vi "Level 3 Climb.vi"() -> ()   [LabVIEW 2018]
uses:
  <vilib>/Rock Robotics/WPI/ThirdParty/Phoenix-LabVIEW/Motor Controller/Controls/CTRE_Phoenix_MotorControl_ControlMode.ctl
  <vilib>/Rock Robotics/WPI/ThirdParty/Phoenix-LabVIEW/Motor Controller/Get/CTRE_Phoenix_MotorController_GetSelectedSensorData.vi
panel:
  in  "Boolean":bool
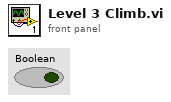
[diagram p1: front panel]
types:
  T1 = typedef "CTRE_Phoenix_MotorControl_ControlMode.ctl" = u16
  T2 = typedef "WPI_MotorControlDeviceRef.ctl" = cluster{"DeviceStatus":errorcluster, "Type":T3, "PWM":cluster{"PWM Channel":T4, "DeadBand":T5}, "CAN":cluster{"Device Number":u8, "SetOutput VI Ref":variant, "GetOutput VI Ref":variant, "Enable VI Ref":variant, "Disable VI Ref":variant, "Data":variant}, "Invert":bool, "DIO PWM":cluster{"PWM \"Enable\" Channel":T4, "DIOChannel":T6, "PWM Rate":dbl}}
  T3 = typedef "WPI_MotorControlType.ctl" = enum16{"PWM", "CAN", "DIO PWM"}
  T4 = typedef "FPGA_DIOPWMChannel.ctl" = enum8{"PWM 0", "PWM 1", "PWM 2", "PWM 3", "PWM 4", "PWM 5", "PWM 6", "PWM 7", "PWM 8", "PWM 9", "PWM MXP 0", "PWM MXP 1", "PWM MXP 2", "PWM MXP 3", "PWM MXP 4", "PWM MXP 5", "PWM MXP 6", "PWM MXP 7", "PWM MXP 8", "PWM MXP 9", "Invalid"}
  T5 = typedef "WPI_PWMDeadband.ctl" = cluster{"Name":string, "maxPositivePwm":i32, "minPositivePwm":i32, "centerPwm":i32, "maxNegativePwm":i32, "minNegativePwm":i32, "angularRange":u16}
  T6 = typedef "FPGA_DIOChannel.ctl" = enum8{"DIO 0", "DIO 1", "DIO 2", "DIO 3", "DIO 4", "DIO 5", "DIO 6", "DIO 7", "DIO 8", "DIO 9", "DIO MXP 0", "DIO MXP 1", "DIO MXP 2", "DIO MXP 3", "DIO MXP 4", "DIO MXP 5", "DIO MXP 6", "DIO MXP 7", "DIO MXP 8", "DIO MXP 9", "DIO MXP 10", "DIO MXP 11", "DIO MXP 12", "DIO MXP 13", "DIO MXP 14", "DIO MXP 15", "SPI Port CS1", "SPI Port CS2", "SPI Port CS3", "SPI Port MISO", "SPI Port MOSI", "Invalid"}
  T7 = typedef "WPI_SwitchDevRef.ctl" = cluster{"DevStatus":errorcluster, "DIO Channel":T6, "CntIndex":T8, "Normally Closed":bool}
  T8 = typedef "FPGA_CounterCtrSystemIndex.ctl" = enum8{"Ctr 0", "Ctr 1", "Ctr 2", "Ctr 3", "Ctr 4", "Ctr 5", "Ctr 6", "Ctr 7", "Invalid"}
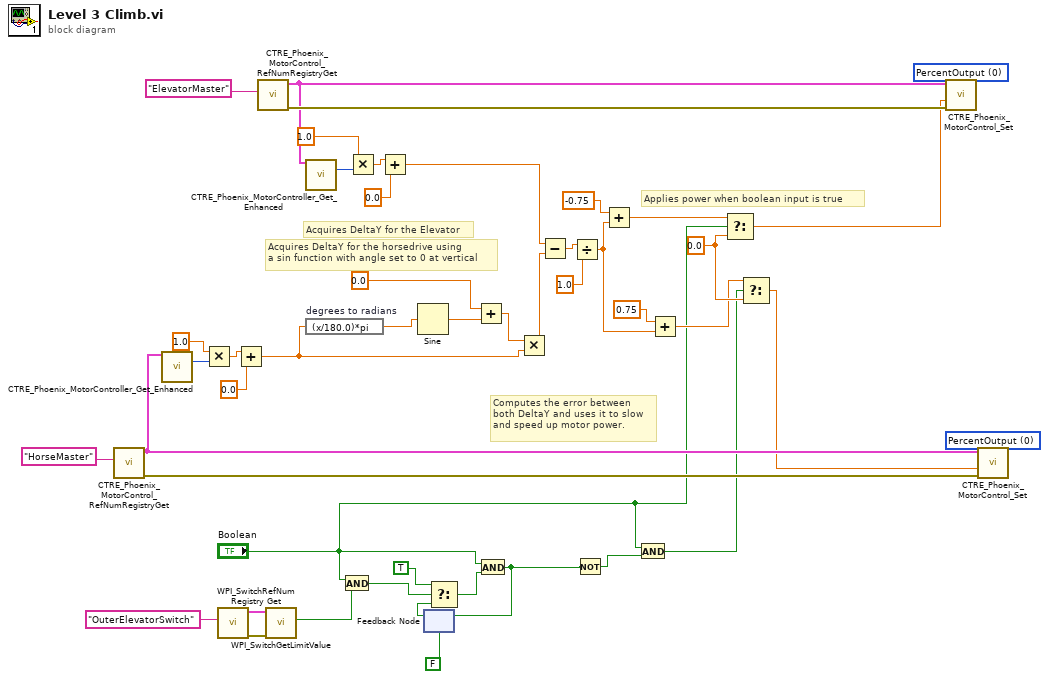
[diagram p0: block diagram]
diagram:
  w42 = T1 0 items=["PercentOutput"=0, "Position"=1, "Velocity"=2, "Current"=3, "Follower"=5, "MotionProfile"=6, "MotionMagic"=7, "MotionProfileArc"=10, "Disabled"=15] ("Control Mode")
  w38 = 0.0 ("f")
  w45 = T1 0 items=["PercentOutput"=0, "Position"=1, "Velocity"=2, "Current"=3, "Follower"=5, "MotionProfile"=6, "MotionMagic"=7, "MotionProfileArc"=10, "Disabled"=15] ("Control Mode")
  # "Applies power when boolean input is true"
  # "Computes the error between\nboth DeltaY and uses it to slow\nand speed up motor power."
  # "Acquires DeltaY for the horsedrive using\na sin function with angle set to 0 at vertical"
  # "Acquires DeltaY for the Elevator"
  n1 = call <vilib>:"CTRE_Phoenix_MotorControl_RefNumRegistryGet.vi"("refnum name"="HorseMaster") -> ("error out"=w41:errorcluster, "PhoenixMotorControlDevRef"=w40:T2)  [unwired: 9 in]
  n2 = call-poly <vilib>:"CTRE_Phoenix_MotorController_Get_Enhanced.vi"("PhoenixMotorControlDevRef"=w40) -> ("Position (Raw Sensor Units)"=w25:i32)  [unwired: 11 in, 3 out]
  n3 = Multiply(x=1.0, y=w25) -> (x*y=w39:dbl)
  n4 = call <vilib>:"WPI_SwitchRefNum Registry Get.vi"("refnum name"="OuterElevatorSwitch") -> ("error out"=w12:errorcluster, "SwitchDevRef"=w11:T7)  [unwired: 9 in]
  n5 = Add(x=w39, y=0.0) -> (x+y=w19:dbl)
  n6 = call <vilib>:"CTRE_Phoenix_MotorControl_RefNumRegistryGet.vi"("refnum name"="ElevatorMaster") -> ("error out"=w46:errorcluster, "PhoenixMotorControlDevRef"=w35:T2)  [unwired: 9 in]
  n7 = call <vilib>:"WPI_SwitchGetLimitValue.vi"("error in (no error)"=w12, "SwitchDevRef"=w11) -> ("Switch Pressed"=w10:bool)  [unwired: 7 in, 2 out]
  n8 = call-poly <vilib>:"CTRE_Phoenix_MotorController_Get_Enhanced.vi"("PhoenixMotorControlDevRef"=w35) -> ("Position (Raw Sensor Units)"=w36:i32)  [unwired: 11 in, 3 out]
  n9 = expression code="(x/180.0)*pi" "degrees to radians"(w19) -> (w21:dbl)
  n10 = And(x="Boolean", y=w10) -> (x .and. y?=w9:bool)
  n11 = Multiply(x=1.0, y=w36) -> (x*y=w37:dbl)
  n12 = Add(x=w37, y=0.0) -> (x+y=w34:dbl)
  n13 = Sine(x=w21) -> (sin(x)=w23:dbl)
  n14 = feedback #1(FALSE) -> (w7:bool)
  n15 = Select(t=TRUE, s=w9, f=w7) -> (s? t:f=w5:bool)
  n16 = Add(x=0.0, y=w23) -> (x+y=w20:dbl)
  n17 = And(x="Boolean", y=w5) -> (x .and. y?=w3:bool)
  n18 = feedback-in #1(w3) -> ()
  n19 = Multiply(x=w20, y=w19) -> (x*y=w24:dbl)
  n20 = Subtract(x=w34, y=w24) -> (x-y=w33:dbl)
  n21 = Divide(x=w33, y=1.0) -> (x/y=w29:dbl)
  n22 = Not(x=w3) -> (.not. x?=w2:bool)
  n23 = Add(x=-0.75, y=w29) -> (x+y=w31:dbl)
  n24 = And(x="Boolean", y=w2) -> (x .and. y?=w1:bool)
  n25 = Add(x=0.75, y=w29) -> (x+y=w28:dbl)
  n26 = Select(t=w31, s="Boolean", f=w38) -> (s? t:f=w27:dbl)
  n27 = Select(t=w28, s=w1, f=w38) -> (s? t:f=w26:dbl)
  n28 = call <vilib>:"CTRE_Phoenix_MotorControl_Set.vi"("error in (no error)"=w46, "Output"=w27, "Control Mode"=w45, "PhoenixMotorControlDevRef"=w35) -> ()  [unwired: 6 in, 2 out]
  n29 = call <vilib>:"CTRE_Phoenix_MotorControl_Set.vi"("error in (no error)"=w41, "Output"=w26, "Control Mode"=w42, "PhoenixMotorControlDevRef"=w40) -> ()  [unwired: 6 in, 2 out]
